vi "8位RGB图像转换为8位灰度图子VI.vi"(11 "path to BMP file":path caption="BMP文件路径") -> (0 "原始图像":picture, 2 "转换后的原始图像":T1(plugin-control), 3 "path":path caption="路径")   [LabVIEW 2018]
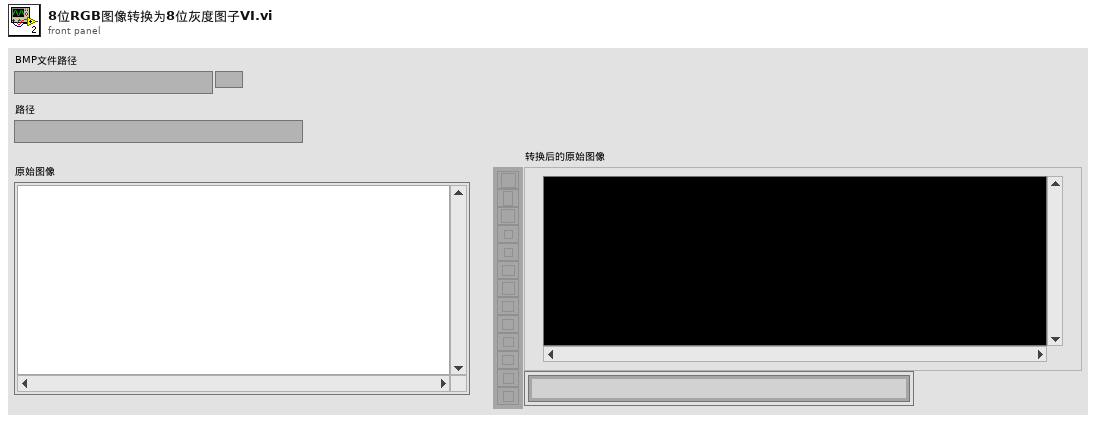
[diagram p1: front panel]
types:
  T1 = typedef "IMAQ Image.ctl" = refnum<image>
  T2 = typedef "imagedata.ctl" = cluster{"image type":i32, "image depth":i32, "image":u8[], "mask":u8[], "colors":u32[], "Rectangle":cluster{"left":i16, "top":i16, "right":i16, "bottom":i16}}
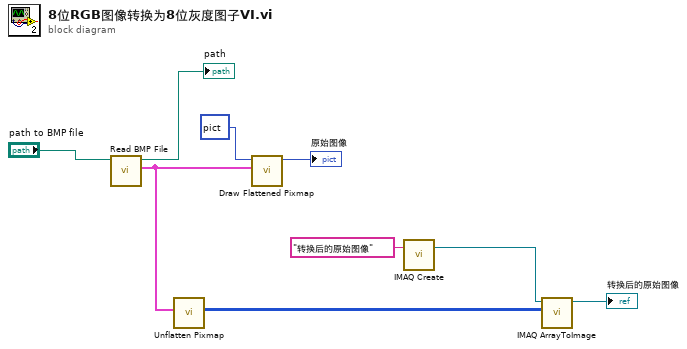
[diagram p0: block diagram]
diagram:
  n1 = call <vilib>:"Read BMP File.vi"("path to BMP file"="path to BMP file") -> ("image data"=w8:T2, "path"=→"path":path)  [unwired: 8 in, 1 out]
  n2 = call <vilib>:"Unflatten Pixmap.vi"("image data"=w8) -> ("8-bit pixmap"=w7:u8[][])  [unwired: 4 in, 6 out]
  n3 = call <vilib>:"Draw Flattened Pixmap.vi"("image data"=w8, "picture"=picture data[5B]) -> ("new picture"=→"原始图像":picture)  [unwired: 7 in]
  n4 = call "IMAQ Create"("Image Name"="转换后的原始图像") -> ("New Image"=w3:T1)  [unwired: 4 in, 1 out]
  n5 = call "IMAQ ArrayToImage"("Image Pixels (U8)"=w7, "Image"=w3) -> ("Image Out"=→"转换后的原始图像":T1)  [unwired: 8 in, 1 out]
